vi "TestRemoteVIServerSend.vi"() -> ()   [LabVIEW 2018]
doc: "MIT License\n\nCopyright (c) 2020 RichardLGP5\n\nPermission is hereby granted, free of charge, to any person obtaining a copy\nof this software and associated documentation files (the \"Software\"), to deal\nin the Software without restriction, including without limitation the rights\nto use, copy, modify, merge, publish, distribute, sublicense, and/or sell\ncopies of the Software, and to permit persons to whom the Software is\nfurnished to do so, subject to the following conditions:\n\nThe above copyright notice and this permission notice shall be included in all\ncopies or substantial portions of the Software.\n\nTHE SOFTWARE IS PROVIDED \"AS IS\", WITHOUT WARRANTY OF ANY KIND, EXPRESS OR\nIMPLIED, INCLUDING BUT NOT LIMITED TO THE WARRANTIES OF MERCHANTABILITY,\nFITNESS FOR A PARTICULAR PURPOSE AND NONINFRINGEMENT. IN NO EVENT SHALL THE\nAUTHORS OR COPYRIGHT HOLDERS BE LIABLE FOR ANY CLAIM, DAMAGES OR OTHER\nLIABILITY, WHETHER IN AN ACTION OF CONTRACT, TORT OR OTHERWISE, ARISING FROM,\nOUT OF OR IN CONNECTION WITH THE SOFTWARE OR THE USE OR OTHER DEALINGS IN THE\nSOFTWARE."
uses:
  MSGR Q Name TypeDef.ctl
panel:
  in  "stop":bool
  in  "Parameters":string
  in  "Msg":string
  in  "MSGR Q name":T1
  in  "Send?":bool
  in  "machine name (\"\":  open local reference)":string
  in  "type specifier VI Refnum (for type only)":refnum<vi>
  out "error out":errorcluster
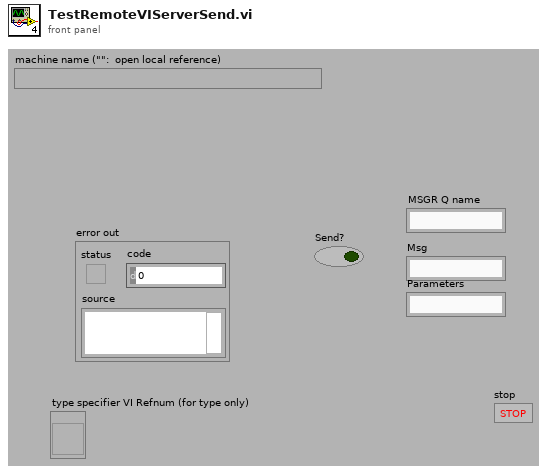
[diagram p1: front panel]
types:
  T1 = typedef "MSGR Q Name TypeDef.ctl" = string
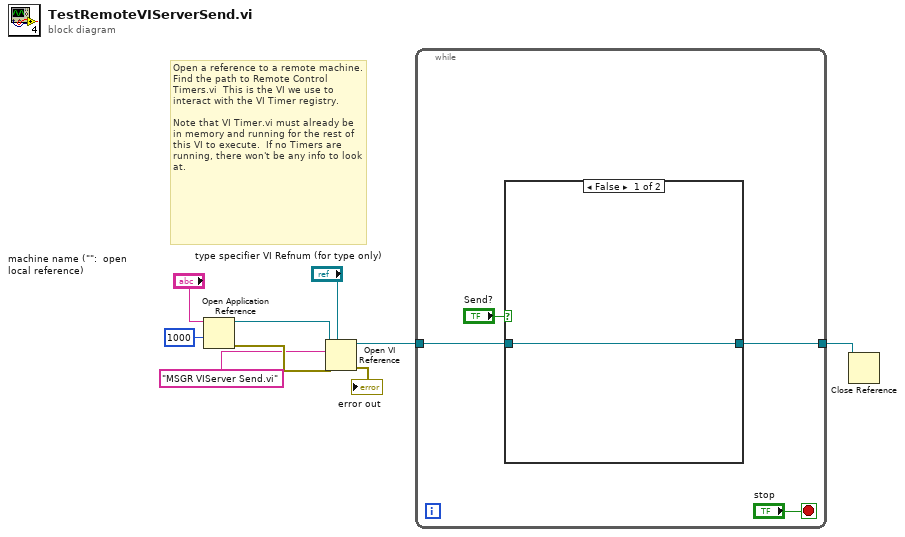
[diagram p0: block diagram]
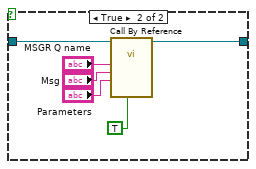
[diagram p2: hidden frame]
diagram:
  # "Open a reference to a remote machine.\nFind the path to Remote Control Timers.vi  This is the VI we use to interact with the VI Timer registry.\n\nNote that VI Timer.vi must already be in memory and running for the rest of this VI to execute.  If no Timers are running, there won't be any info to look at."
  n1 = Open Application Reference(9:1000 ("timeout ms (60000)"), 11:"machine name (\"\":  open local reference)") -> (0:w8:errorcluster, 3:w5:refnum<vi>)  [unwired: 1 in, 1 out]
  n2 = Open VI Reference(type specifier VI Refnum (for type only)="type specifier VI Refnum (for type only)", application reference (local)=w5, vi path="MSGR VIServer Send.vi", error in (no error)=w8) -> (vi reference=w2:refnum<vi>, error out=→"error out":errorcluster)  [unwired: 2 in]
  n3 = while {
    tunnel: w2 -> [w12]
    tunnel: [w10] -> w1
    stop <- "stop" stop-if-true
    n4 = case shown="False" "Send?" {
      tunnel: w12 -> [w14 w20]
      tunnel: [w14 w15] -> w10
      frame False {
      }
      frame True {
        n5 = call-by-ref "?"(reference=w20, "Write?"=TRUE, "Parameters"="Parameters", "Msg"="Msg", "MSGR Q name"="MSGR Q name") -> (reference out=w15:refnum<vi>)  [unwired: 9 in, 1 out]
      }
    }
  }
  n6 = Close Reference(reference=w1) -> ()  [unwired: 1 in, 1 out]
